vi "Destroy Linked List.vi"(8 "error in (no error)":errorcluster, 11 "Linked List Ref":refnum<data-value>) -> (0 "error out":errorcluster)   [LabVIEW 2020, in "Linked Lists.lvlib" / "Linked List Ref.lvclass"]
uses:
  <vilib>/gpm_packages/@cs/linked-list/Source/Linked List/Linked List Ref/Linked List Ref.lvclass
  <vilib>/gpm_packages/@cs/linked-list/Source/Linked List/ILinkedList/ILinked List.lvclass
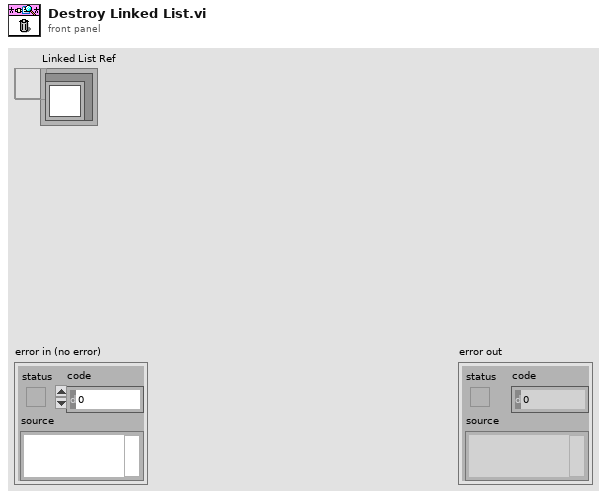
[diagram p1: front panel]
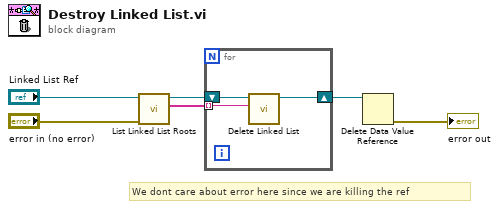
[diagram p0: block diagram]
diagram:
  # "We dont care about error here since we are killing the ref"
  n1 = call <vilib>:"List Linked List Roots.vi"("error in (no error)"="error in (no error)", "Linked List Ref"="Linked List Ref") -> ("Root IDs"=w1:string[], "Linked List Ref out"=w3:refnum<data-value>)  [unwired: 6 in, 2 out]
  n2 = for {
    shift-right: [w8] -> w2
    shift-left: w3 -> [w9]
    tunnel: w1 -> [w7] mode=indexing
    n3 = call <vilib>:"Delete Linked List.vi"("Linked List ID"=w7, "Linked List Ref"=w9) -> ("Linked List Ref out"=w8:refnum<data-value>)  [unwired: 8 in, 1 out]
  }
  n4 = Delete Data Value Reference(data value reference=w2) -> (error out=→"error out":errorcluster)  [unwired: 1 in, 1 out]
